vi "Get Gabor Coefficients.vi"(8 "error in (no error)":errorcluster, 11 "RefNum in":T1) -> (0 "error out":errorcluster, 2 "coefficients":cdb[][](array[numeric]) format="%.2f", 3 "RefNum out":T1)   [LabVIEW 2017, in "SoundVib_Gabor.lvlib"]
doc: "Returns a complex array, <B>coefficients</B>, containing the Gabor coefficients from the stored data block referenced by <B>RefNum in</B>. Each row in <B>coefficients</B> contains the spectrum in a window."
uses:
  <vilib>/addons/Sound and Vibration/Order Analysis/Gabor Order Tracking/SoundVib_Gabor.lvlib
  <vilib>/addons/Sound and Vibration/Order Analysis/Ref Gabor Order Tracking/GT RefNum.ctl
  <resource>/sndvib.dll
panel:
  # "Get Gabor Coefficients"
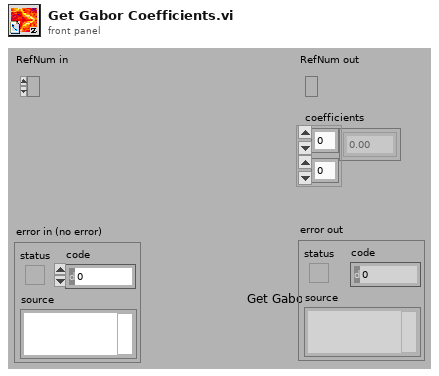
[diagram p1: front panel]
types:
  T1 = typedef "SoundVib_Gabor.lvlib/GT RefNum.ctl" = refnum<k1>
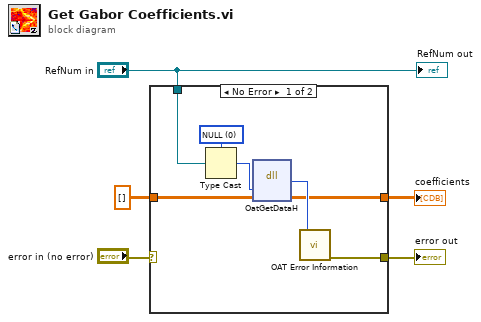
[diagram p0: block diagram]
diagram:
  n1 = case shown="No Error" "error in (no error)" {
    selector: "error in (no error)" -> [_ w14]
    tunnel: [w12 w14] -> w5
    tunnel: [w7 w13] -> w3
    tunnel: "RefNum in" -> [w8 _]
    tunnel: cdb[][] [] ("hGraphArray") -> [w6 w13]
    frame No Error {
      w11 = u32 0 items=["NULL"]
      n2 = Type Cast(type=w11, x=w8) -> (*(type *) &x=w10:u32)
      n3 = dll-call lib="C:/Program Files (x86)/National Instruments/LabVIEW 2017/resource/sndvib.*" fn="OatGetDataH"("Ref In"=w10, "Coefficients"=w6) -> ("return type"=w9:i32, "Coefficients"=w7:cdb[][])  [unwired: 4 in, 2 out]
      n4 = call <vilib>:"OAT Error Information.vi"("error code"=w9) -> ("error out"=w12:errorcluster)  [unwired: 6 in]
    }
    frame Error {
    }
  }
  "error out" <- w5
  "coefficients" <- w3
  "RefNum out" <- "RefNum in"
